vi "Is Read Only.vi"(8 "error in":errorcluster, 11 "Filesystem Statistics in":refnum<class "Filesystem Statistics.lvclass">) -> (0 "error out":errorcluster, 2 "read only?":bool, 3 "Filesystem Statistics out":refnum<class "Filesystem Statistics.lvclass">)   [LabVIEW 2020, in "NI_SFTP.lvlib" / "Filesystem Statistics.lvclass"]
doc: "Returns TRUE if this Filesystem Statistics object represents a read-only filesystem.\n\nRead-only filesystems contains files whose attributes indicate they are writable. However, no files can be modified, created, renamed, or deleted."
uses:
  <vilib>/net/SFTP/Filesystem Statistics/Filesystem Statistics.lvclass
  <vilib>/net/SFTP/Filesystem Statistics/Filesystem Statistics.lvclass/Filesystem Statistics.ctl
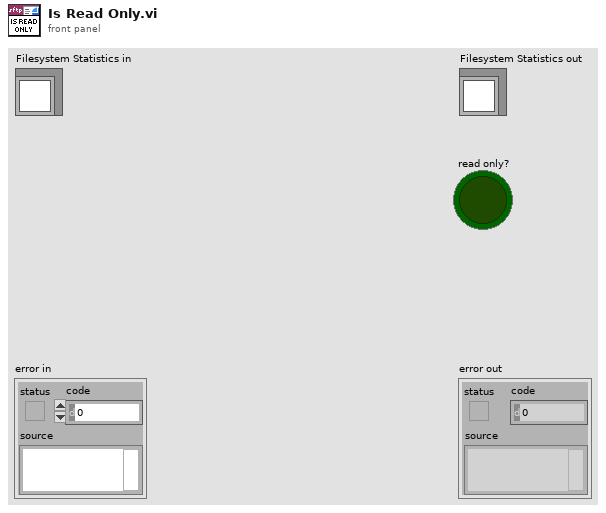
[diagram p1: front panel]
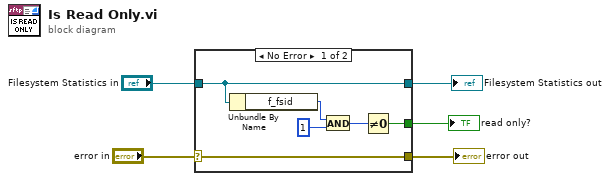
[diagram p0: block diagram]
diagram:
  n1 = case shown="No Error" "error in" {
    selector: "error in" -> [w11 w13]
    tunnel: [w11 w13] -> w2
    tunnel: [w10 w12] -> w3
    tunnel: "Filesystem Statistics in" -> [w10 w12]
    tunnel: [w6 _] -> w1
    frame No Error {
      n2 = Unbundle By Name(w10) -> ("f_fsid"=w9:u64)
      n3 = And(x=w9, y=u64 1) -> (x .and. y?=w7:u64)
      n4 = Not Equal To 0?(x=w7) -> (x != 0?=w6:bool)
    }
    frame Error {
    }
  }
  "error out" <- w2
  "Filesystem Statistics out" <- w3
  "read only?" <- w1
